vi "prompt - frame added.vi"() -> (3 "message":string="PayloadID field cannot \nbe empty. Frame was\nnot added.")   [LabVIEW 2020, in "FrameEditor.lvlib"]
uses:
  FrameEditor.lvlib
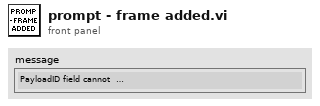
[diagram p1: front panel]
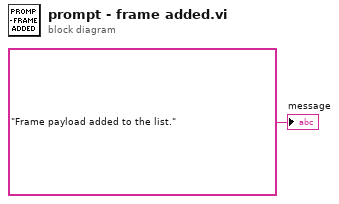
[diagram p0: block diagram]
diagram:
  "message" <- "Frame payload added to the list." ("message")
